vi "AH2500.AVERAGE.vi"(7 "error in (no error)":errorcluster, 9 "Sample Time (s)":T1(ring), 10 "VISA resource name":refnum<visa-resource-name>) -> (0 "error out":errorcluster, 1 "Read out result":string, 2 "Send string":string, 3 "VISA resource name out":refnum<visa-resource-name>)   [LabVIEW 2019, in "Inst.AH2500.lvclass"]
uses:
  Inst.AH2500.lvclass
panel:
  # "Average over time: setting the measurement time"
  # "Default setting is 4"
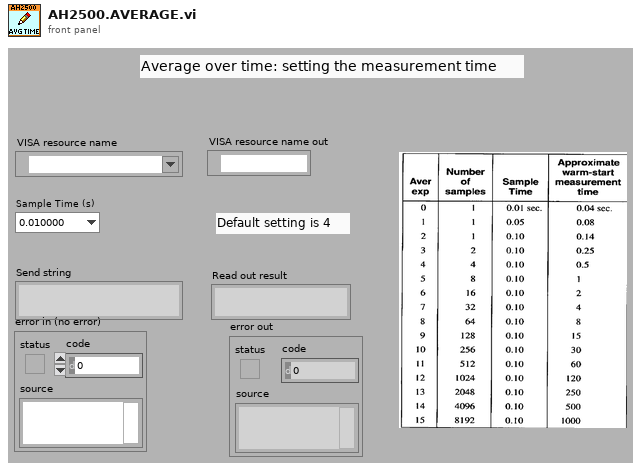
[diagram p1: front panel]
types:
  T1 = enum16{"0.010000", "0.050000", "0.100000", "0.200000", "0.400000", "0.800000", "1.600000", "3.200000", "6.400000", "12.800000", "25.600000", "51.200000", "102.400000", "204.800000", "409.600000", "819.200000"}
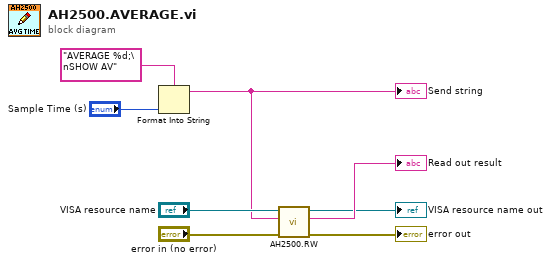
[diagram p0: block diagram]
diagram:
  n1 = Format Into String(format string="AVERAGE %d;\nSHOW AV", "Sample Time (s)") -> (resulting string=w5:string)  [unwired: 2 in, 1 out]
  "Send string" <- w5
  n2 = call "AH2500.RW.vi"("error in (no error)"="error in (no error)", "write buffer"=w5, "VISA Refnum in"="VISA resource name") -> ("error out"=→"error out":errorcluster, "read buffer"=→"Read out result":string, "VISA Refnum out"=→"VISA resource name out":refnum<visa-resource-name>)  [unwired: 6 in]
